vi "GetCurrAD.vi"(0 "data0":u8, 1 "data1":u8, 2 "data2":u8, 3 "data3":u8, 4 "data4":u8, 5 "data5":u8, 6 "data6":u8, 7 "data7":u8, 8 "类型":u32(ring)=4 items=["PCI5121"=1, "PCI9810"=2, "USBCAN1"=3, "USBCAN2"=4, "PCI9820"=5, "CAN232"=6, "PCI5110"=7, "CANLite(mini)"=8, "ISA9620"=9, "ISA5420"=10, "PC104CAN"=11, "CANET"=17, "DNP9810"=13, "USBCAN-E-U"=20, "USBCAN-2E-U"=21], 9 "ID Receive":i32=10, 10 "设备索引":u32(ring) items=["0", "1", "2", "3", "4", "5", "6", "7", "8", "9", "10", "11", "12", "13", "14", "15", ""], 12 "CAN路数":u32(ring) items=["0", "1"], 14 "ExternFlag":u8, 16 "ID Send":u32, 18 "DataLen":u8) -> (20 "发送状态":bool, 21 "Data":u8[](array[numeric]), 22 "Value":u64)   [LabVIEW 2013]
uses:
  BHN01/AutoBurn/Settings/ControlCAN.dll
panel:
  in  "设备索引 2":u32(ring) items=["0", "1", "2", "3", "4", "5", "6", "7", "8", "9", "10", "11", "12", "13", "14", "15", ""]
  in  "CAN路数 2":u32(ring) items=["0", "1"]
  in  "类型 2":u32(ring)=4 items=["PCI5121"=1, "PCI9810"=2, "USBCAN1"=3, "USBCAN2"=4, "PCI9820"=5, "CAN232"=6, "PCI5110"=7, "CANLite(mini)"=8, "ISA9620"=9, "ISA5420"=10, "PC104CAN"=11, "CANET"=17, "DNP9810"=13, "USBCAN-E-U"=20, "USBCAN-2E-U"=21]
  out "VCI_CAN_OBJ_T":T1 {"ID" format="%x"}
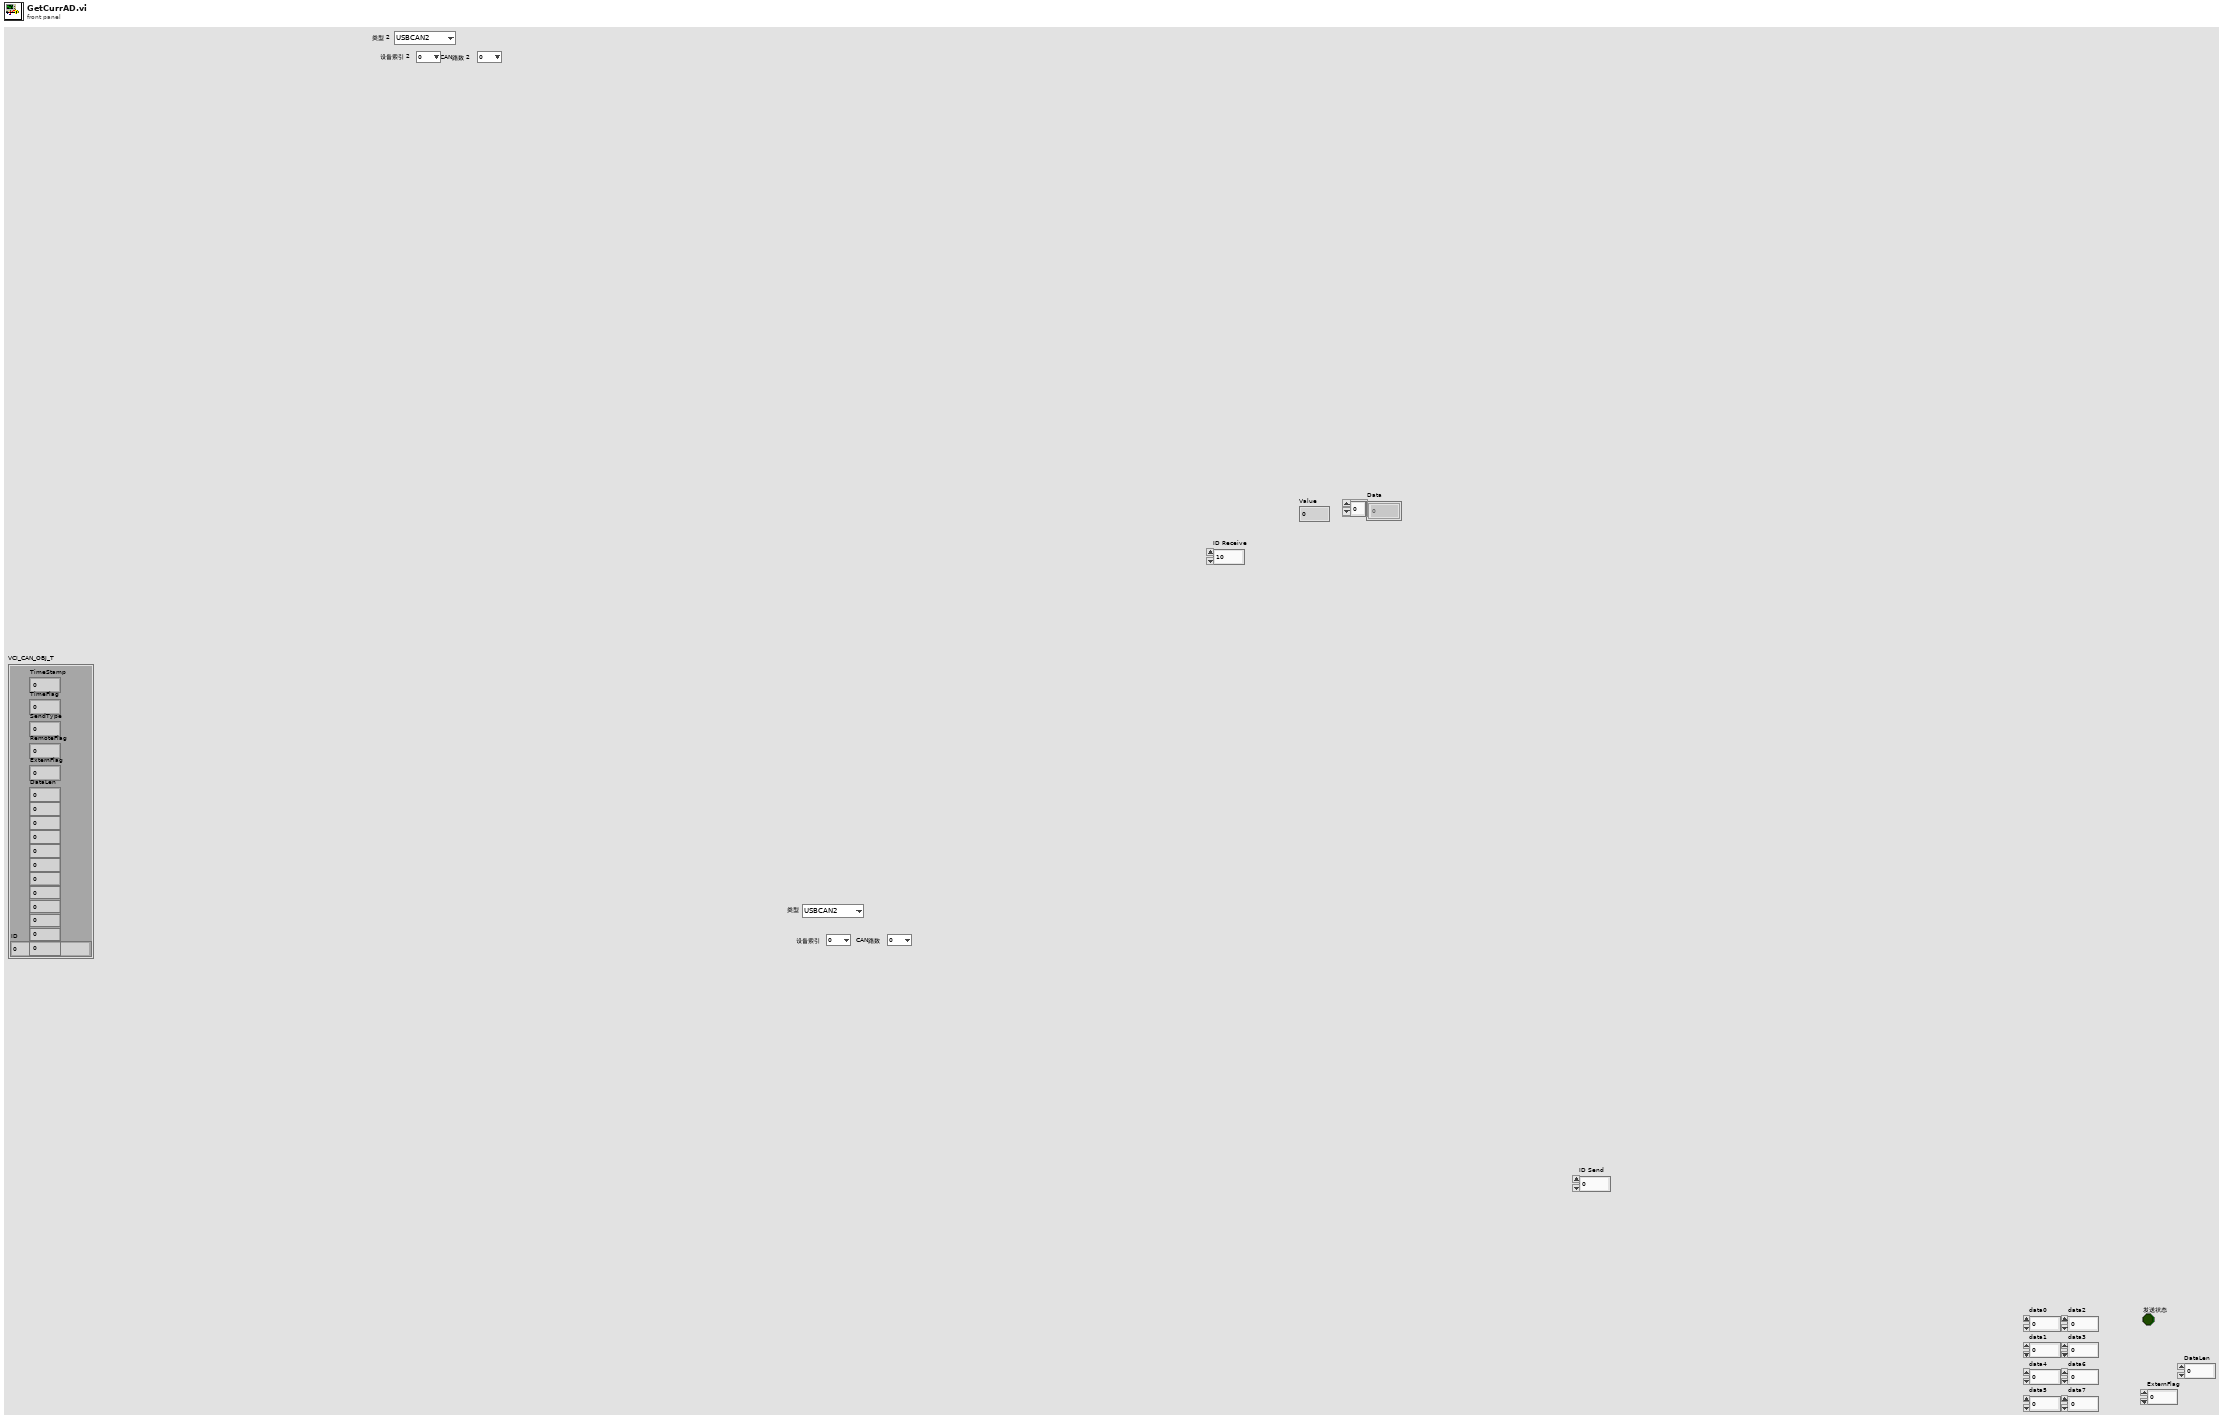
[diagram p1: front panel]
types:
  T1 = cluster{"ID":u32, "TimeStamp":u32, "TimeFlag":u8, "SendType":u8, "RemoteFlag":u8, "ExternFlag":u8, "DataLen":u8, u8, u8, u8, u8, u8, u8, u8, u8, u8, u8, u8}
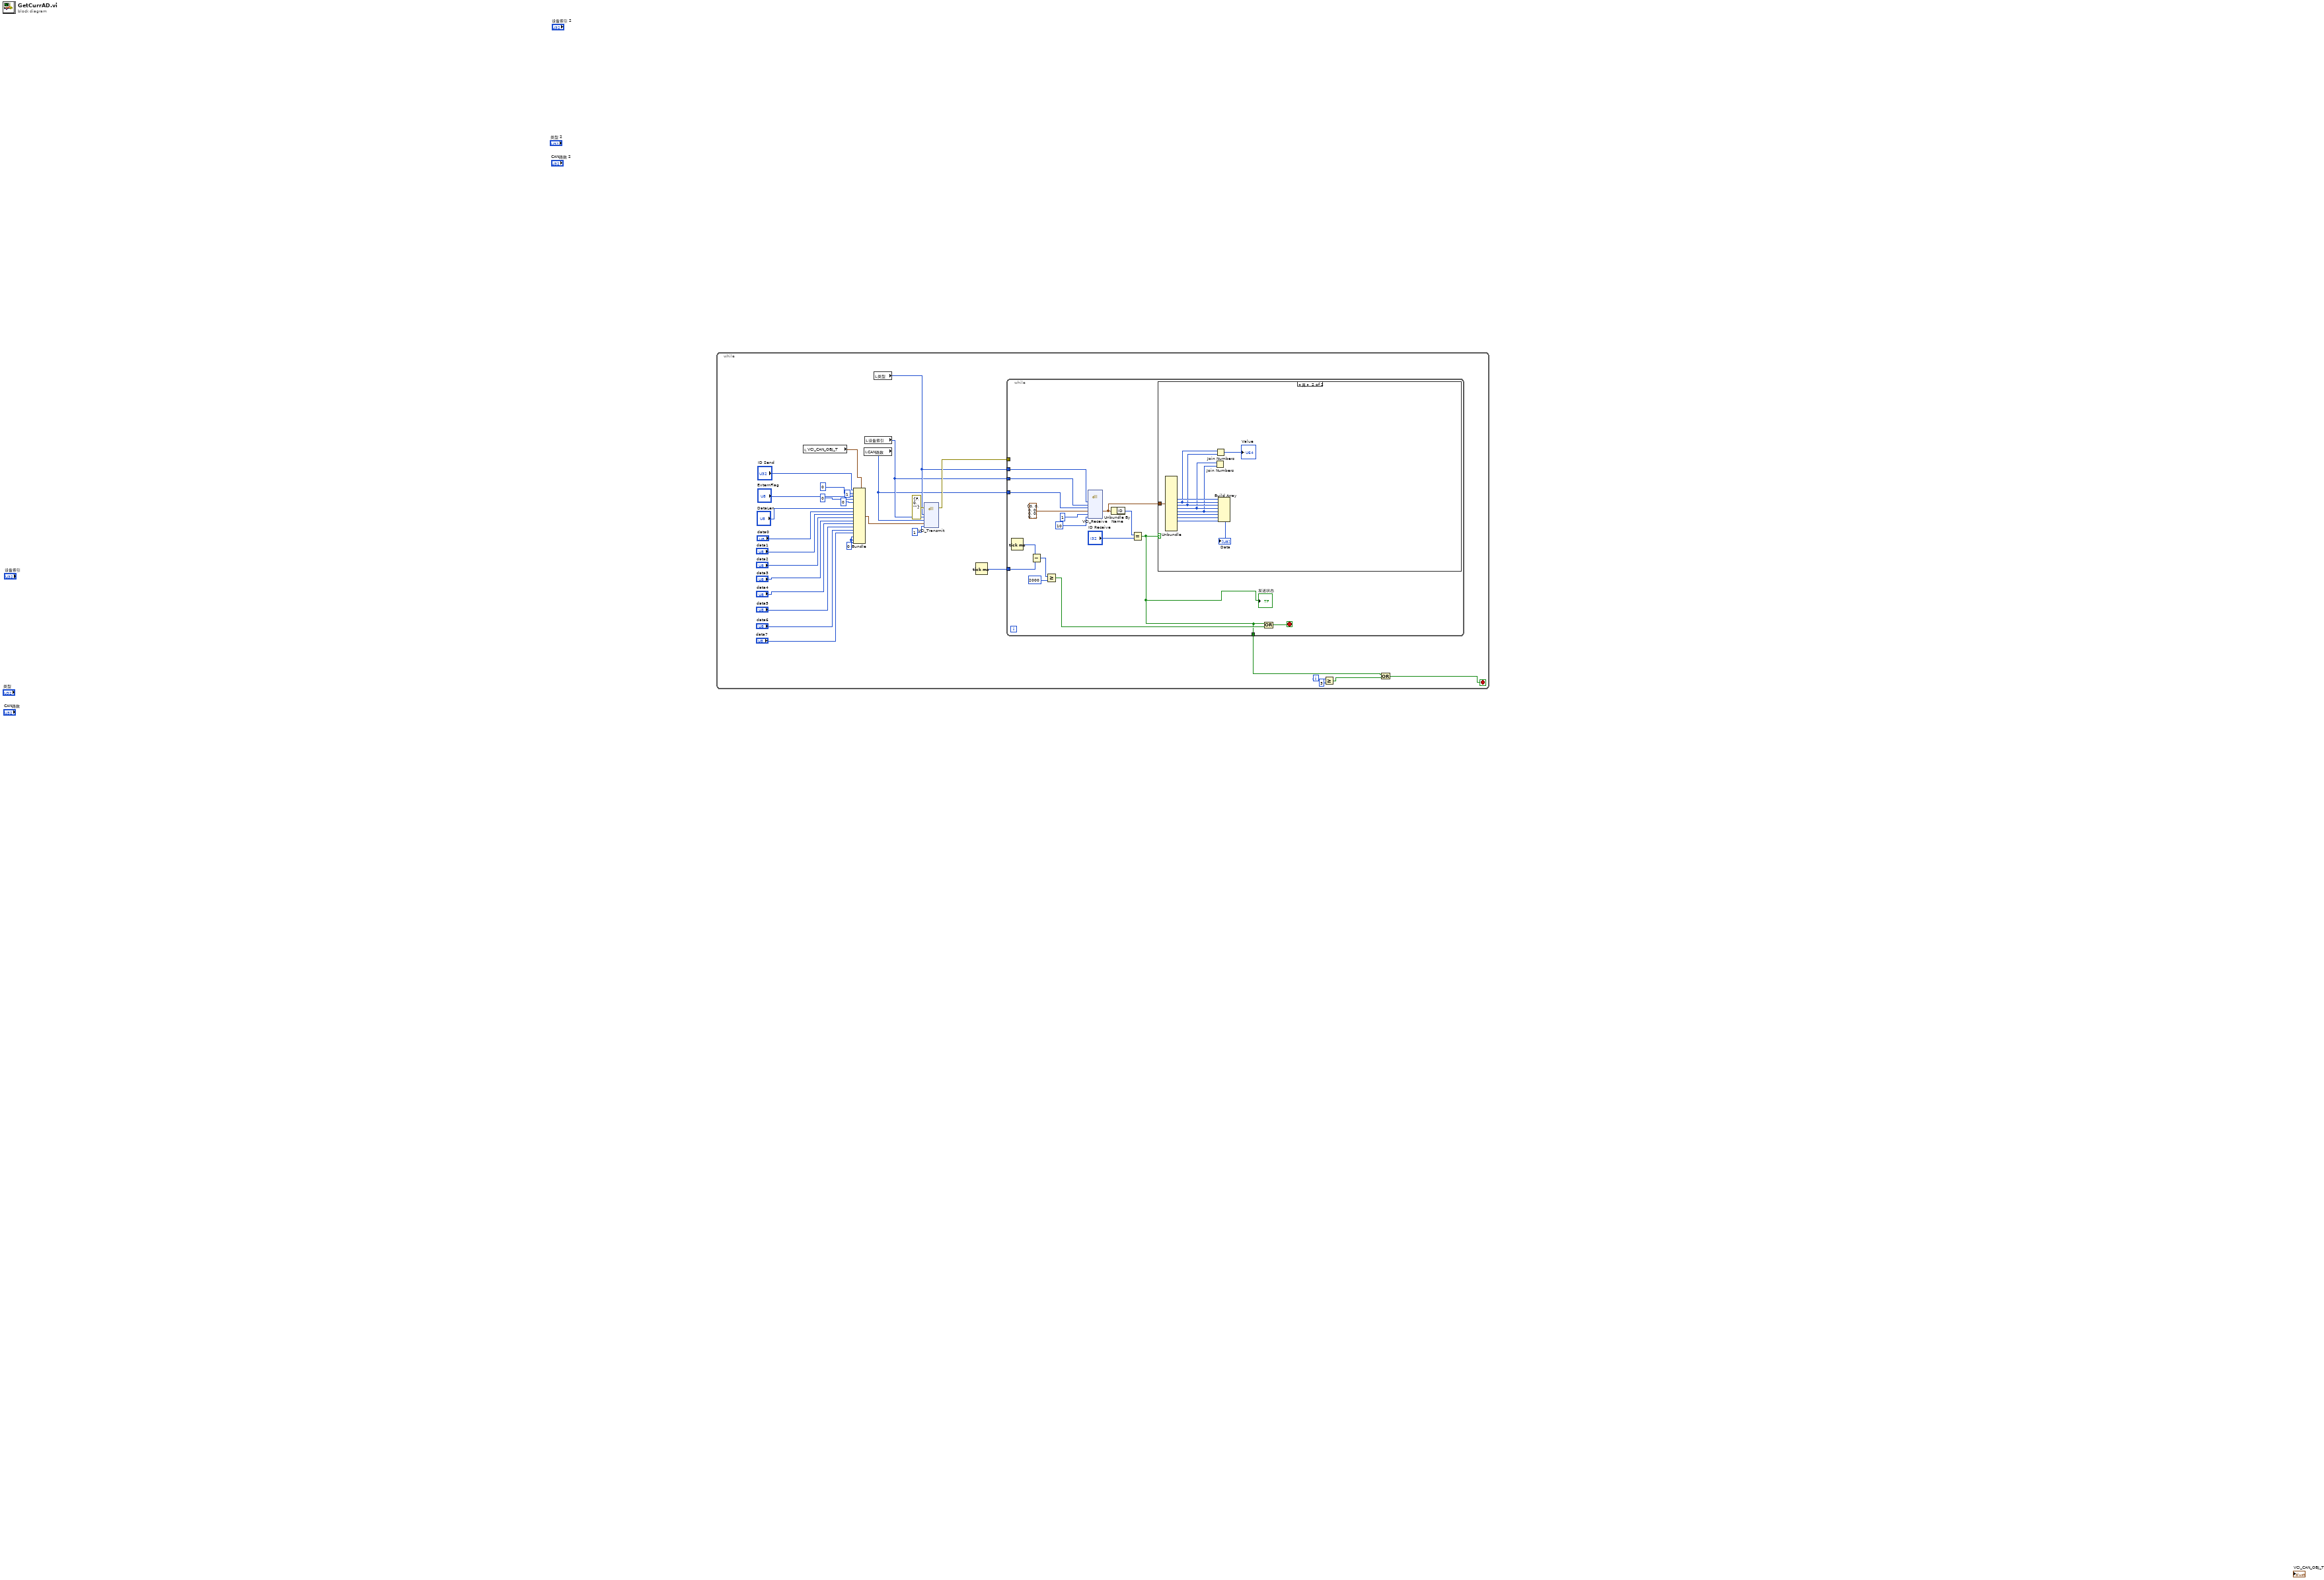
[diagram p0: block diagram]
diagram:
  n1 = while {
    i -> [w3]
    stop <- w4 stop-if-true
    w24 = u8 0 ("元素")
    n2 = local read "VCI_CAN_OBJ_T"() -> (w28:T1)
    n3 = Bundle(cluster=w28, "ID"="ID Send", "TimeStamp"=u8 0 ("RemoteFlag"), "TimeFlag"=u8 1, "SendType"=u8 0 ("DataLen"), "RemoteFlag"=u8 0, "ExternFlag"="ExternFlag", "DataLen"="DataLen", "data0", "data1", "data2", "data3", "data4", "data5", "data6", "data7", w24, w24, w24) -> (w29:T1)
    n4 = local read "CAN路数"() -> (w6:u32)
    n5 = local read "设备索引"() -> (w7:u32)
    n6 = local read "类型"() -> (w8:u32)
    n7 = dll-call lib="F:/Bluewave New Energy/SVN_Work/AutoTest_TestStand/trunk/AutoTest_TestStand/Driver/ZlgCan/BHN01/AutoBurn/Settings/ControlCAN.dll" fn="VCI_Transmit"(error in=errorcluster {"status"=FALSE, "code"=0, "source"=""} ("错误输入（无错误）"), "DeviceType"=w8, "DeviceInd"=w7, "CANInd"=w6, "pSend"=w29, "Len"=u32 1) -> (error out=w9:errorcluster)  [unwired: 4 in, 5 out]
    n8 = Tick Count (ms)() -> (millisecond timer value=w10:u32)
    n9 = while {
      tunnel: w10 -> [w42]
      tunnel: w9 -> [_]
      tunnel: w8 -> [w35]
      tunnel: w7 -> [w34]
      tunnel: w6 -> [w33]
      tunnel: [w31] -> w5
      stop <- w37 stop-if-true
      n10 = Tick Count (ms)() -> (millisecond timer value=w43:u32)
      n11 = Subtract(x=w43, y=w42) -> (x-y=w41:u32)
      n12 = Greater Or Equal?(x=w41, y=u32 2000) -> (x >= y?=w38:bool)
      n13 = dll-call lib="F:/Bluewave New Energy/SVN_Work/AutoTest_TestStand/trunk/AutoTest_TestStand/Driver/ZlgCan/BHN01/AutoBurn/Settings/ControlCAN.dll" fn="VCI_Receive"("DeviceType"=w35, "DeviceInd"=w34, "CANInd"=w33, "pReceive"=T1 {"ID"=0, "TimeStamp"=0, "TimeFlag"=0, "SendType"=0, "RemoteFlag"=0, "ExternFlag"=0, "DataLen"=0, 0, 0, 0, 0, 0, 0, 0, 0, 0, 0, 0}, "Len"=u32 1, "WaitTime"=10) -> ("pReceive"=w36:T1)  [unwired: 8 in, 3 out]
      n14 = Unbundle By Name(w36) -> ("ID"=w40:u32)
      n15 = Equal?(x=w40, y="ID Receive") -> (x = y?=w31:bool)
      "发送状态" <- w31
      n16 = case shown="真" w31 {
        tunnel: w36 -> [_ w57]
        frame False {
        }
        frame True {
          n17 = Unbundle(w57) -> (w55:u8, w51:u8, w50:u8, w49:u8, w48:u8, w54:u8, w53:u8, w52:u8)  [unwired: 10 out]
          n18 = Join Numbers(hi=w49, lo=w48) -> ()  [unwired: 1 out]
          n19 = Join Numbers(hi=w51, lo=w50) -> ((hi.lo)=→"Value":u16)
          n20 = Build Array(w55, w51, w50, w49, w48, w54, w53, w52) -> (→"Data":u8[])
        }
      }
      n21 = Or(x=w31, y=w38) -> (x .or. y?=w37:bool)
    }
    n22 = Greater Or Equal?(x=w3, y=3) -> (x >= y?=w1:bool)
    n23 = Or(x=w5, y=w1) -> (x .or. y?=w4:bool)
  }
